vi "_MPI_I_v2.vi"(9 "MPI_I":T1={"wait(ms)"=300, "Start"=22.5, "Stop"=23.5, "Step"=0.005, "save"=FALSE, "file_name"="LP_914.0_Tmin_100519.csv"} {"Step" format="%#.6f"; "Stop" format="%.2f"; "Start" format="%.2f"}, 10 "Control":T3={"GPIB_ATT"="28", "6501Dev#"=1, "GPIB_SP"="18", "GPIB_PM"="13", "GPIB_DSA"="11", "GPIB_DMM (TPD)"="23", "GPIB_MPI"="2", "mortor設定"=[{"Axis"=0, "ID"=0, "HIspeed"=200.0, "LOspeed"=100.0, "ACCEL(ms)"=100.0, "Sratio"=50.0, "フリーラン\n"=FALSE, "文字列"="DSB HOT/COLD"}, {"Axis"=1, "ID"=0, "HIspeed"=4.0, "LOspeed"=4.0, "ACCEL(ms)"=100.0, "Sratio"=50.0, "フリーラン\n"=TRUE, "文字列"="SubMM Att"}], "DATAパス"=path "C:/Documents and Settings/?澤佳?/デスクトップ/data/プロトカ?トリッジ/100811_protC4-5/100814_WCA_P0", "DBパス "=path "Z:/band10/Labview_ALMA/MIX95/test", "comment"="NOLO", "ColdCarts"="003601", "Th"=295.0, "Tc"=77.0, "Set_SIS_volt"=1.9086021505376345, "Offset"=0.0, "control"=0, "FreqLO"=850.0, "Set_Mag_Cur"=800.0, "MPI offset(mm)"=22.99, "HOT/COLD"=0} {"HOT/COLD" items=["DSB", "SBR", "GainComp"]; "control" items=["CLOSE LOOP", "OPEN LOOP", "Not Control"]}, 11 "Bias_LO_equip":T2={"Node address"=19, "CAN Interface"="CAN0", "Cartridge band"=10, "Slave Node in"={"Address"=19, "Serial Number"=[16, 71, 55, 76, 1, 8, 0, -15]}, "ObjHandle out"=89653312, "POL"=0, "sb"=1, "GPIB_SM (SIS S,V)"="24", "GPIB_DMM (SIS I)"="22", "GPIB_SM (MAG I) "="25", "GPIB_SG(LO)"="19", "GPIB_PW (PAMP) "="6", "GPIB_TMP1(8ch)"="12", "GPIB_TMP2(2ch)  "="13", "WCA_avg"=10, "Rsen"=10.0, "BiasModule"=1, "LOModule "=2, "WCA_LO_FREQ_SET"={"YTO Low freq. [GHz]"=14.41, "YTO High freq. [GHz]"=17.71, "Kvco"=1, "Lock Pol."=0, "SET LO FREQ"=94.44444, "Multiplier"=6.0, "YTO (HEX)"=1650, "YTO ( FREQ)"=15.73967, "NULL PLL INTEGRATOR"=FALSE}, "Res for"=0} {"Res for" items=["none", "series res", "parallel res"]; "WCA_LO_FREQ_SET"."YTO ( FREQ)" min=25 max=150 step=0.0001 format="%.3f"; "WCA_LO_FREQ_SET"."Multiplier" min=3 max=6 step=3; "WCA_LO_FREQ_SET"."SET LO FREQ" min=25 max=150 step=0.0001 format="%.3f"; "WCA_LO_FREQ_SET"."Lock Pol." items=["Lower", "Upper"]; "WCA_LO_FREQ_SET"."Kvco" items=["7.5MHz/V", "15MHz/V"]; "WCA_LO_FREQ_SET"."YTO High freq. [GHz]" format="%.3f"; "WCA_LO_FREQ_SET"."YTO Low freq. [GHz]" format="%.3f"; "LOModule" items=["Manual Gunn+PAMP"=0, "B10Lab LO"=1, "WCA LO"=2, ""=3, "YIG発信器"=4, "none"=99]; "BiasModule" items=["B10Lab Bias"=0, "WCA BiasModule"=1, "none"=99]; "Slave Node in"."Serial Number" format="%.0x"; "Slave Node in"."Address" format="%.0x"; "Cartridge band" max=10 step=1; "Node address" format="%.0x"}) -> ()   [LabVIEW 2017]
uses:
  __sub_vi/WCA_NAOJ_sub_vi/WCA_Global.vi
panel:
  out "Link済み":bool
  out "測定結果":string="22.500000\t0.005734\t-22.415552\t0.000000\r\n22.505000\t0.005523\t-22.578525\t0.000000\r\n22.510000\t0.005256\t-22.793438\t0.000000\r\n22.515000\t0.004945\t-23.058715\t0.000000\r\n22.520000\t0.004614\t-23.359281\t0.000000\r\n22.525000\t0.004245\t-23.721315\t0.000000\r\n22.530000\t0.003864\t-24.129460\t0.000000\r\n22.535000\t0.003450\t-24.621406\t0.000000\r\n22.540000\t0.003079\t-25.115677\t0.000000\r\n22.545000\t0.002679\t-25.719949\t0.000000\r\n22.550000\t0.002300\t-26.383666\t0.000000\r\n22.555000\t0.001984\t-27.025021\t0.000000\r\n22.560000\t0.001693\t-27.714380\t0.000000\r\n22.565000\t0.001475\t-28.311933\t0.000000\r\n22.570000\t0.001304\t-28.845892\t0.000000\r\n22.575000\t0.001222\t-29.128293\t0.000000\r\n22.580000\t0.001212\t-29.166372\t0.000000\r\n22.585000\t0.001271\t-28.957383\t0.000000\r\n22.590000\t0.001431\t-28.442633\t0.000000\r\n22.595000\t0.001655\t-27.811233\t0.000000\r\n22.600000\t0.001956\t-27.086156\t0.000000\r\n22.605000\t0.002292\t-26.397778\t0.000000\r\n22.610000\t0.002688\t-25.706144\t0.000000\r\n22.615000\t0.003103\t-25.082714\t0.000000\r\n22.620000\t0.003504\t-24.554793\t0.000000\r\n22.625000\t0.003921\t-24.066386\t0.000000\r\n22.630000\t0.004307\t-23.658483\t0.000000\r\n22.635000\t0.004688\t-23.290559\t0.000000\r\n22.640000\t0.005010\t-23.001943\t0.000000\r\n22.645000\t0.005315\t-22.745237\t0.000000\r\n22.650000\t0.005559\t-22.550104\t0.000000\r\n22.655000\t0.005750\t-22.403450\t0.000000\r\n22.660000\t0.005904\t-22.288183\t0.000000\r\n22.665000\t0.005977\t-22.235167\t0.000000\r\n22.670000\t0.006021\t-22.203508\t0.000000\r\n22.675000\t0.005971\t-22.239813\t0.000000\r\n22.680000\t0.005879\t-22.307054\t0.000000\r\n22.685000\t0.005762\t-22.394599\t0.000000\r\n22.690000\t0.005562\t-22.547604\t0.000000\r\n22.695000\t0.005314\t-22.746111\t0.000000\r\n22.700000\t0.005045\t-22.971535\t0.000000\r\n22.705000\t0.004723\t-23.258069\t0.000000\r\n22.710000\t0.004380\t-23.584902\t0.000000\r\n22.715000\t0.003999\t-23.980996\t0.000000\r\n22.720000\t0.003634\t-24.396426\t0.000000\r\n22.725000\t0.003244\t-24.888549\t0.000000\r\n22.730000\t0.002855\t-25.443665\t0.000000\r\n22.735000\t0.002502\t-26.016867\t0.000000\r\n22.740000\t0.002148\t-26.679556\t0.000000\r\n22.745000\t0.001837\t-27.359807\t0.000000\r\n22.750000\t0.001603\t-27.950556\t0.000000\r\n22.755000\t0.001401\t-28.534193\t0.000000\r\n22.760000\t0.001287\t-28.903067\t0.000000\r\n22.765000\t0.001249\t-29.034584\t0.000000\r\n22.770000\t0.001293\t-28.885123\t0.000000\r\n22.775000\t0.001419\t-28.481615\t0.000000\r\n22.780000\t0.001606\t-27.941896\t0.000000\r\n22.785000\t0.001865\t-27.292257\t0.000000\r\n22.790000\t0.002177\t-26.621715\t0.000000\r\n22.795000\t0.002520\t-25.985512\t0.000000\r\n22.800000\t0.002894\t-25.385645\t0.000000\r\n22.805000\t0.003295\t-24.821960\t0.000000\r\n22.810000\t0.003703\t-24.314346\t0.000000\r\n22.815000\t0.004088\t-23.884753\t0.000000\r\n22.820000\t0.004465\t-23.502155\t0.000000\r\n22.825000\t0.004812\t-23.176455\t0.000000\r\n22.830000\t0.005132\t-22.896888\t0.000000\r\n22.835000\t0.005395\t-22.680359\t0.000000\r\n22.840000\t0.005624\t-22.499570\t0.000000\r\n22.845000\t0.005806\t-22.360968\t0.000000\r\n22.850000\t0.005909\t-22.285051\t0.000000\r\n22.855000\t0.005994\t-22.222782\t0.000000\r\n22.860000\t0.005983\t-22.230520\t0.000000\r\n22.865000\t0.005947\t-22.256918\t0.000000\r\n22.870000\t0.005828\t-22.345036\t0.000000\r\n22.875000\t0.005688\t-22.450427\t0.000000\r\n22.880000\t0.005489\t-22.605447\t0.000000\r\n22.885000\t0.005227\t-22.817301\t0.000000\r\n22.890000\t0.004955\t-23.049353\t0.000000\r\n22.895000\t0.004608\t-23.365309\t0.000000\r\n22.900000\t0.004244\t-23.722410\t0.000000\r\n22.905000\t0.003861\t-24.133058\t0.000000\r\n22.910000\t0.003472\t-24.594641\t0.000000\r\n22.915000\t0.003099\t-25.087196\t0.000000\r\n22.920000\t0.002722\t-25.651342\t0.000000\r\n22.925000\t0.002351\t-26.288028\t0.000000\r\n22.930000\t0.002026\t-26.932620\t0.000000\r\n22.935000\t0.001711\t-27.668109\t0.000000\r\n22.940000\t0.001488\t-28.274409\t0.000000\r\n22.945000\t0.001329\t-28.764979\t0.000000\r\n22.950000\t0.001235\t-29.083049\t0.000000\r\n22.955000\t0.001236\t-29.079323\t0.000000\r\n22.960000\t0.001311\t-28.824636\t0.000000\r\n22.965000\t0.001457\t-28.365643\t0.000000\r\n22.970000\t0.001681\t-27.744581\t0.000000\r\n22.975000\t0.001948\t-27.105136\t0.000000\r\n22.980000\t0.002277\t-26.426160\t0.000000\r\n22.985000\t0.002634\t-25.793183\t0.000000\r\n22.990000\t0.003033\t-25.180846\t0.000000\r\n22.995000\t0.003423\t-24.656451\t0.000000\r\n23.000000\t0.003821\t-24.177673\t0.000000\r\n23.005000\t0.004204\t-23.762980\t0.000000\r\n23.010000\t0.004588\t-23.383444\t0.000000\r\n23.015000\t0.004937\t-23.065272\t0.000000\r\n23.020000\t0.005233\t-22.812866\t0.000000\r\n23.025000\t0.005521\t-22.580200\t0.000000\r\n23.030000\t0.005715\t-22.430119\t0.000000\r\n23.035000\t0.005871\t-22.312576\t0.000000\r\n23.040000\t0.005956\t-22.250694\t0.000000\r\n23.045000\t0.006003\t-22.216606\t0.000000\r\n23.050000\t0.005987\t-22.228198\t0.000000\r\n23.055000\t0.005918\t-22.278001\t0.000000\r\n23.060000\t0.005795\t-22.369750\t0.000000\r\n23.065000\t0.005607\t-22.512764\t0.000000\r\n23.070000\t0.005359\t-22.708782\t0.000000\r\n23.075000\t0.005074\t-22.946812\t0.000000\r\n23.080000\t0.004747\t-23.235570\t0.000000\r\n23.085000\t0.004389\t-23.576443\t0.000000\r\n23.090000\t0.004015\t-23.963653\t0.000000\r\n23.095000\t0.003599\t-24.438700\t0.000000\r\n23.100000\t0.003204\t-24.943143\t0.000000\r\n23.105000\t0.002808\t-25.515642\t0.000000\r\n23.110000\t0.002409\t-26.180983\t0.000000\r\n23.115000\t0.002071\t-26.837654\t0.000000\r\n23.120000\t0.001760\t-27.545318\t0.000000\r\n23.125000\t0.001510\t-28.209512\t0.000000\r\n23.130000\t0.001326\t-28.775449\t0.000000\r\n23.135000\t0.001216\t-29.151093\t0.000000\r\n23.140000\t0.001179\t-29.286520\t0.000000\r\n23.145000\t0.001232\t-29.094316\t0.000000\r\n23.150000\t0.001361\t-28.661642\t0.000000\r\n23.155000\t0.001550\t-28.097496\t0.000000\r\n23.160000\t0.001817\t-27.405447\t0.000000\r\n23.165000\t0.002117\t-26.742545\t0.000000\r\n23.170000\t0.002484\t-26.048449\t0.000000\r\n23.175000\t0.002880\t-25.406512\t0.000000\r\n23.180000\t0.003273\t-24.850182\t0.000000\r\n23.185000\t0.003695\t-24.324361\t0.000000\r\n23.190000\t0.004106\t-23.865536\t0.000000\r\n23.195000\t0.004509\t-23.458793\t0.000000\r\n23.200000\t0.004870\t-23.124791\t0.000000\r\n23.205000\t0.005193\t-22.845750\t0.000000\r\n23.210000\t0.005451\t-22.635087\t0.000000\r\n23.215000\t0.005665\t-22.468384\t0.000000\r\n23.220000\t0.005870\t-22.313360\t0.000000\r\n23.225000\t0.005967\t-22.242141\t0.000000\r\n23.230000\t0.006016\t-22.206582\t0.000000\r\n23.235000\t0.006012\t-22.209666\t0.000000\r\n23.240000\t0.005954\t-22.252247\t0.000000\r\n23.245000\t0.005851\t-22.327588\t0.000000\r\n23.250000\t0.005663\t-22.469197\t0.000000\r\n23.255000\t0.005452\t-22.634234\t0.000000\r\n23.260000\t0.005178\t-22.858254\t0.000000\r\n23.265000\t0.004861\t-23.132404\t0.000000\r\n23.270000\t0.004524\t-23.444438\t0.000000\r\n23.275000\t0.004140\t-23.829587\t0.000000\r\n23.280000\t0.003752\t-24.257187\t0.000000\r\n23.285000\t0.003333\t-24.771647\t0.000000\r\n23.290000\t0.002933\t-25.326820\t0.000000\r\n23.295000\t0.002558\t-25.921657\t0.000000\r\n23.300000\t0.002193\t-26.589911\t0.000000\r\n23.305000\t0.001874\t-27.272420\t0.000000\r\n23.310000\t0.001612\t-27.927508\t0.000000\r\n23.315000\t0.001391\t-28.567384\t0.000000\r\n23.320000\t0.001259\t-29.001330\t0.000000\r\n23.325000\t0.001181\t-29.278678\t0.000000\r\n23.330000\t0.001190\t-29.243509\t0.000000\r\n23.335000\t0.001283\t-28.917496\t0.000000\r\n23.340000\t0.001438\t-28.423257\t0.000000\r\n23.345000\t0.001672\t-27.766676\t0.000000\r\n23.350000\t0.001953\t-27.093267\t0.000000\r\n23.355000\t0.002296\t-26.389714\t0.000000\r\n23.360000\t0.002671\t-25.733798\t0.000000\r\n23.365000\t0.003065\t-25.135284\t0.000000\r\n23.370000\t0.003477\t-24.587966\t0.000000\r\n23.375000\t0.003885\t-24.105553\t0.000000\r\n23.380000\t0.004277\t-23.688699\t0.000000\r\n23.385000\t0.004638\t-23.336252\t0.000000\r\n23.390000\t0.004990\t-23.018612\t0.000000\r\n23.395000\t0.005273\t-22.779365\t0.000000\r\n23.400000\t0.005526\t-22.576009\t0.000000\r\n23.405000\t0.005727\t-22.420402\t0.000000\r\n23.410000\t0.005863\t-22.318890\t0.000000\r\n23.415000\t0.005958\t-22.249134\t0.000000\r\n23.420000\t0.005993\t-22.223557\t0.000000\r\n23.425000\t0.005980\t-22.232843\t0.000000\r\n23.430000\t0.005879\t-22.307054\t0.000000\r\n23.435000\t0.005750\t-22.403450\t0.000000\r\n23.440000\t0.005575\t-22.537621\t0.000000\r\n23.445000\t0.005324\t-22.737399\t0.000000\r\n23.450000\t0.005051\t-22.966029\t0.000000\r\n23.455000\t0.004738\t-23.244361\t0.000000\r\n23.460000\t0.004385\t-23.580670\t0.000000\r\n23.465000\t0.004017\t-23.961338\t0.000000\r\n23.470000\t0.003605\t-24.430983\t0.000000\r\n23.475000\t0.003231\t-24.907155\t0.000000\r\n23.480000\t0.002822\t-25.494245\t0.000000\r\n23.485000\t0.002465\t-26.082148\t0.000000\r\n23.490000\t0.002135\t-26.705513\t0.000000\r\n23.495000\t0.001804\t-27.438718\t0.000000\r\n23.500000\t0.001571\t-28.038128\t0.000000\r\n" caption="スプレッドシート文字列"
  out "XYグラフ":cluster{dbl[], dbl[]}(graph)
  # "POWER(dBm ) -5～２０ｄBm"
  # "LO freq. [GHz]"
  # "YTO LOW\n/High Freq."
  # "ZERO Intgrtr"
  # "Node Address"
  # "Serial Number"
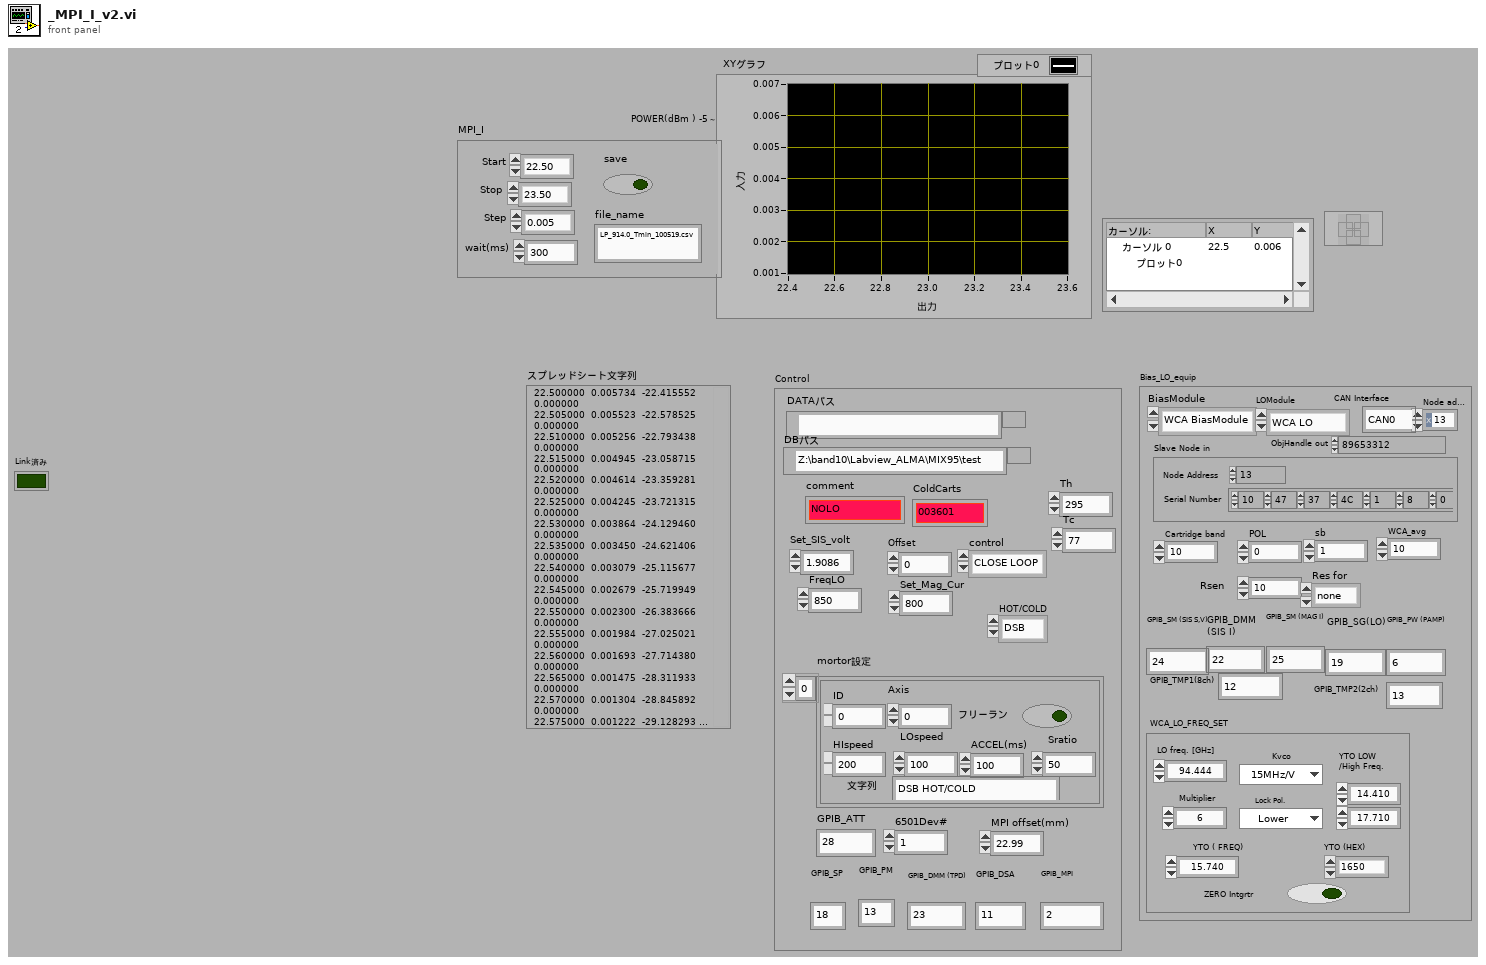
[diagram p1: front panel]
types:
  T1 = cluster{"wait(ms)":i32, "Start":dbl, "Stop":dbl, "Step":dbl, "save":bool, "file_name":string}
  T2 = cluster{"Node address":u16, "CAN Interface":string, "Cartridge band":u32, "Slave Node in":cluster{"Address":i16, "Serial Number":i8[]}, "ObjHandle out":u32, "POL":u32, "sb":u32, "GPIB_SM (SIS S,V)":string, "GPIB_DMM (SIS I)":string, "GPIB_SM (MAG I) ":string, "GPIB_SG(LO)":string, "GPIB_PW (PAMP) ":string, "GPIB_TMP1(8ch)":string, "GPIB_TMP2(2ch)  ":string, "WCA_avg":i32, "Rsen":dbl, "BiasModule":u16, "LOModule ":u16, "WCA_LO_FREQ_SET":cluster{"YTO Low freq. [GHz]":sgl, "YTO High freq. [GHz]":sgl, "Kvco":u16, "Lock Pol.":u16, "SET LO FREQ":sgl, "Multiplier":sgl, "YTO (HEX)":u16, "YTO ( FREQ)":sgl, "NULL PLL INTEGRATOR":bool}, "Res for":u16}
  T3 = cluster{"GPIB_ATT":string, "6501Dev#":i16, "GPIB_SP":string, "GPIB_PM":string, "GPIB_DSA":string, "GPIB_DMM (TPD)":string, "GPIB_MPI":string, "mortor設定":cluster{"Axis":i16, "ID":i16, "HIspeed":dbl, "LOspeed":dbl, "ACCEL(ms)":dbl, "Sratio":dbl, "フリーラン\n":bool, "文字列":string}[], "DATAパス":path, "DBパス ":path, "comment":string, "ColdCarts":string, "Th":dbl, "Tc":dbl, "Set_SIS_volt":dbl, "Offset":dbl, "control":u16, "FreqLO":dbl, "Set_Mag_Cur":dbl, "MPI offset(mm)":dbl, "HOT/COLD":u16}
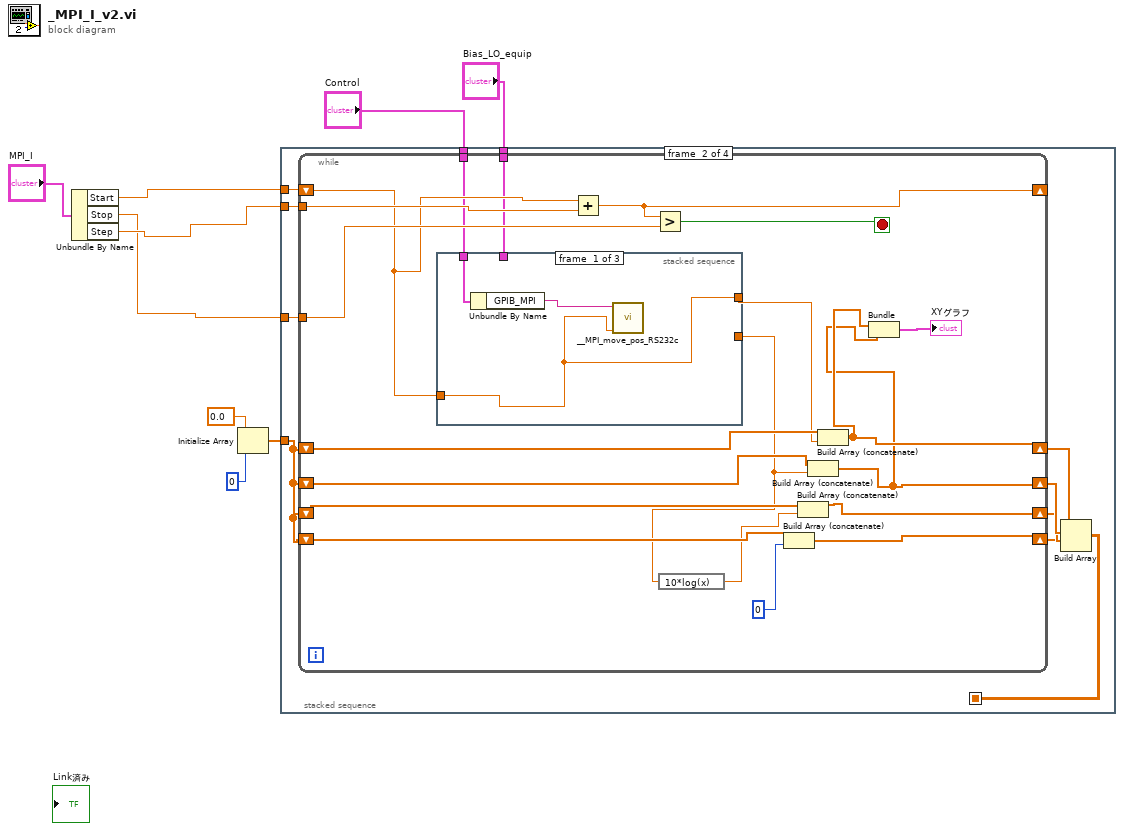
[diagram p0: block diagram]
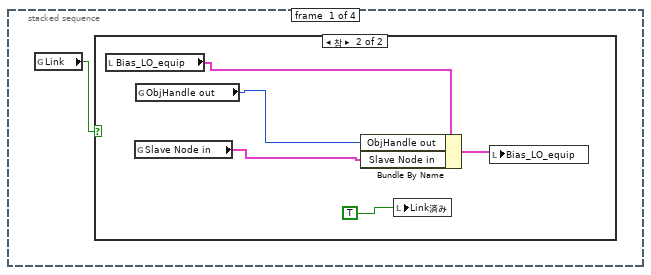
[diagram p2: hidden frame]
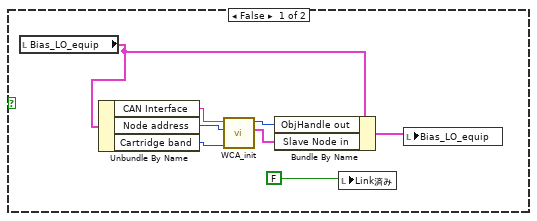
[diagram p3: hidden frame]
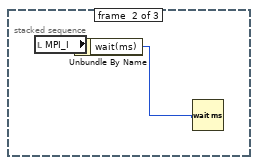
[diagram p4: hidden frame]
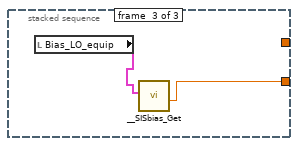
[diagram p5: hidden frame]
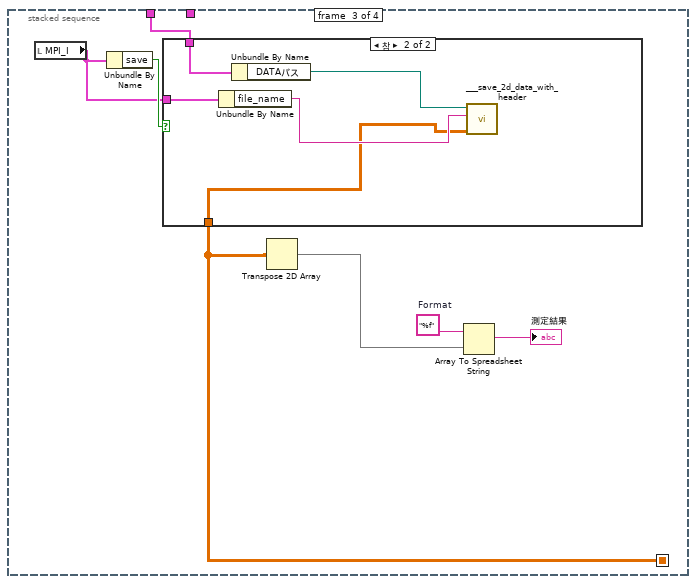
[diagram p6: hidden frame]
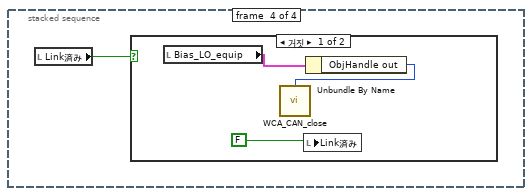
[diagram p8: hidden frame]
diagram:
  n1 = Unbundle By Name("MPI_I") -> ("Start"=w3:dbl, "Stop"=w1:dbl, "Step"=w2:dbl)
  n2 = Initialize Array(0.0, 0) -> (w7:dbl[])
  n3 = stacked-sequence {
    seq-local: [_ w26 _ _] -> [_ _ w62 _]
    tunnel: w3 -> [_ w34 _ _]
    tunnel: w2 -> [_ w33 _ _]
    tunnel: w1 -> [_ w32 _ _]
    tunnel: w7 -> [_ w31 _ _]
    tunnel: "Control" -> [_ w25 w64 _]
    tunnel: "Bias_LO_equip" -> [_ w24 _ _]
    frame #0 {
      n4 = global read "WCA_Global.vi" "Link"() -> (w10:bool)
      n5 = case shown="참" w10 {
        frame False {
          n6 = local read "Bias_LO_equip"() -> (w12:T2)
          n7 = Unbundle By Name(w12) -> ("CAN Interface"=w16:string, "Node address"=w15:u16, "Cartridge band"=w14:u32)
          n8 = call "WCA_init.vi"("Cartridge band"=w14, "Node address"=w15, "CAN Interface"=w16) -> ("Slave Node in"=w17:cluster{"Address":i16, "Serial Number":i8[]}, "ObjHandle out"=w18:u32)  [unwired: 4 in, 3 out]
          n9 = Bundle By Name(cluster=w12, "ObjHandle out"=w18, "Slave Node in"=w17) -> (w13:T2)
          n10 = local write "Link済み"(FALSE) -> ()
          n11 = local write "Bias_LO_equip"(w13) -> ()
        }
        frame True {
          n12 = local read "Bias_LO_equip"() -> (w22:T2)
          n13 = global read "WCA_Global.vi" "Slave Node in"() -> (w20:cluster{"Address":i16, "Serial Number":i8[]})
          n14 = global read "WCA_Global.vi" "ObjHandle out"() -> (w21:u32)
          n15 = Bundle By Name(cluster=w22, "ObjHandle out"=w21, "Slave Node in"=w20) -> (w23:T2)
          n16 = local write "Link済み"(TRUE) -> ()
          n17 = local write "Bias_LO_equip"(w23) -> ()
        }
      }
    }
    frame #1 {
      n18 = while {
        shift-right: [w50] -> _
        shift-left: w34 -> [w51]
        tunnel: w33 -> [w54]
        tunnel: w32 -> [w52]
        shift-right: [w41] -> w30
        shift-left: w31 -> [w49]
        shift-right: [w40] -> w29
        shift-left: w31 -> [w47]
        shift-right: [w42] -> w28
        shift-left: w31 -> [w46]
        shift-right: [w43] -> w27
        shift-left: w31 -> [w45]
        tunnel: w25 -> [w36]
        tunnel: w24 -> [w35]
        stop <- w53 stop-if-true
        n19 = stacked-sequence {
          tunnel: w51 -> [w57 _ _]
          tunnel: [w57 _ _] -> w48
          tunnel: [_ _ w61] -> w38
          tunnel: w36 -> [w56 _ _]
          tunnel: w35 -> [_ _ _]
          frame #0 {
            n20 = Unbundle By Name(w56) -> ("GPIB_MPI"=w55:string)
            n21 = call "__MPI_move_pos_RS232c.vi"("pos"=w57, "VISAリソース名"=w55) -> ()  [unwired: 5 in, 1 out]
          }
          frame #1 {
            n22 = local read "MPI_I"() -> (w59:T1)
            n23 = Unbundle By Name(w59) -> ("wait(ms)"=w58:i32)
            n24 = Wait (ms)(milliseconds to wait=w58) -> ()  [unwired: 1 out]
          }
          frame #2 {
            n25 = local read "Bias_LO_equip"() -> (w60:T2)
            n26 = call "__SISbias_Get.vi"("Bias_LO_equip"=w60) -> ("Get_I(uA)"=w61:dbl)  [unwired: 8 in, 2 out]
          }
        }
        n27 = Add(x=w51, y=w54) -> (x+y=w50:dbl)
        n28 = Greater?(x=w50, y=w52) -> (0:w53:bool)
        n29 = expression code="10*log(x)"(w38) -> (w37:dbl)
        n30 = Build Array (concatenate)(w45, 0) -> (w43:dbl[])
        n31 = Build Array (concatenate)(w46, w37) -> (w42:dbl[])
        n32 = Build Array (concatenate)(w47, w38) -> (w40:dbl[])
        n33 = Build Array (concatenate)(w49, w48) -> (w41:dbl[])
        n34 = Bundle(w41, w40) -> (→"XYグラフ":cluster{dbl[], dbl[]})  [unwired: 1 in]
      }
      n35 = Build Array(w30, w29, w28, w27) -> (w26:dbl[][])
    }
    frame #2 {
      w68 = "%f"  # Format
      n36 = local read "MPI_I"() -> (w63:T1)
      n37 = Unbundle By Name(w63) -> ("save"=w65:bool)
      n38 = case shown="참" w65 {
        tunnel: w64 -> [_ w73]
        tunnel: w63 -> [_ w71]
        tunnel: w62 -> [_ w69]
        frame False {
        }
        frame True {
          n39 = Unbundle By Name(w71) -> ("file_name"=w70:string)
          n40 = Unbundle By Name(w73) -> ("DATAパス"=w72:path)
          n41 = call "___save_2d_data_with_header.vi"("配列"=w69, "file_name"=w70, "パス"=w72) -> ()  [unwired: 8 in, 1 out]
        }
      }
      n42 = Transpose 2D Array(2D array=w62) -> (transposed array=w66:dbl[][])
      n43 = Array To Spreadsheet String(array=w66, 3:w68) -> (spreadsheet string=→"測定結果":string)  [unwired: 1 in]
    }
    frame #3 {
      n44 = local read "Link済み"() -> (w74:bool)
      n45 = case shown="거짓" w74 {
        frame False {
          n46 = local read "Bias_LO_equip"() -> (w76:T2)
          n47 = local write "Link済み"(FALSE) -> ()
          n48 = Unbundle By Name(w76) -> ("ObjHandle out"=w75:u32)
          n49 = call "WCA_CAN_close.vi"("ObjHandle in"=w75) -> ()  [unwired: 14 in, 1 out]
        }
        frame True {
        }
      }
    }
  }
